vi "DAQmx Reference Trigger (Analog Window).vi"(0 "task/channels in":refnum<k21>, 1 "when":i32(ring)=10163 items=["Entering Window"=10163, "Leaving Window"=10208], 5 "source":string, 7 "window top":dbl=0.5 format="%0.2f", 9 "window bottom":dbl format="%0.2f", 11 "error in":errorcluster, 12 "pretrigger samples per channel":u32=500) -> (4 "task out":refnum<k21>, 15 "error out":errorcluster)   [LabVIEW 2011]
doc: "Configures the task to stop the acquisition when the device acquires all pretrigger samples; an analog signal enters or leaves a range you specify; and the device acquires all post-trigger samples. When you use a Reference Trigger, the default for the read RelativeTo property is <B>First Pretrigger Sample</B> with a read Offset of 0."
uses:
  C:/Program Files/National Instruments/LabVIEW 2011/resource/objmgr/daqmx.rc
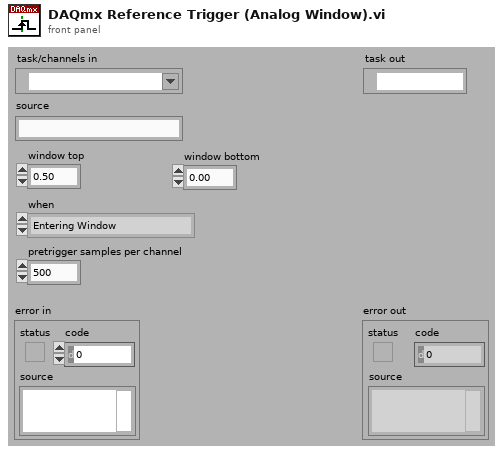
[diagram p1: front panel]
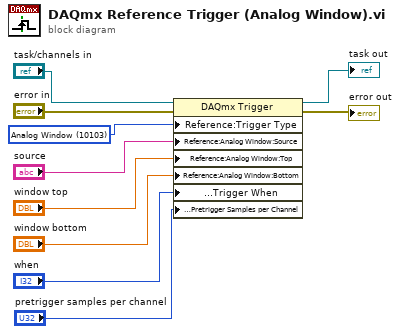
[diagram p0: block diagram]
diagram:
  w7 = 10103 items=["Analog Edge"=10099, "Digital Edge"=10150, "Analog Window"=10103, "None"=10230] ("Start:Trigger Type")
  n1 = property class="DAQmx Trigger"(reference="task/channels in", error in="error in", "Reference:Trigger Type"=w7, "Reference:Analog Window:Source"="source", "Reference:Analog Window:Top"="window top", "Reference:Analog Window:Bottom"="window bottom", "Reference:Analog Window:Trigger When"="when", "Reference:Pretrigger Samples per Channel"="pretrigger samples per channel") -> (reference out=→"task out":refnum<k21>, error out=→"error out":errorcluster)
